vi "ArrayToExcel.vi"() -> ()   [LabVIEW 2020]
uses:
  <vilib>/Analysis/NI_AALBase.lvlib
panel:
  out "F-format string":string[][](array[string])
  out "Waveform Graph":dbl[][](graph)
  # "Diego Jáuregui Ontiveros\nCarlos Uriel Casas Casas\nAlejandro López González"
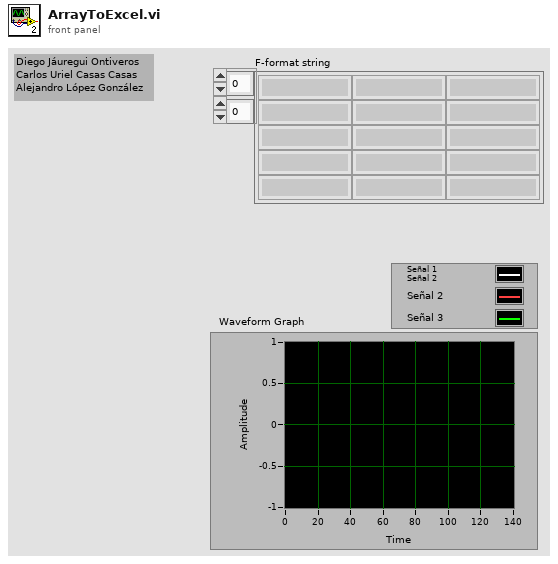
[diagram p1: front panel]
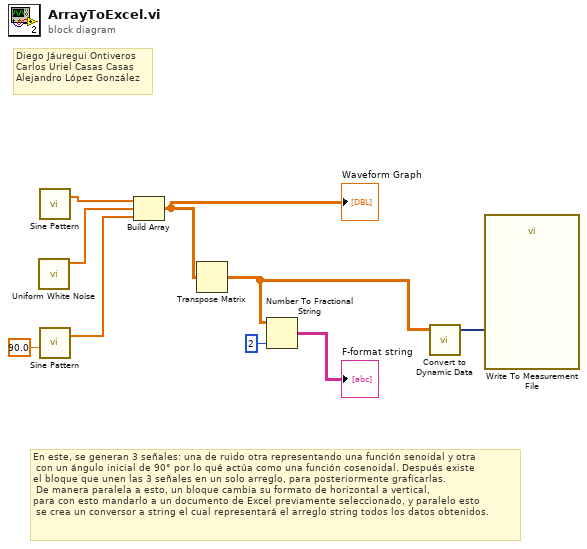
[diagram p0: block diagram]
diagram:
  # "En este, se generan 3 señales: una de ruido otra representando una función senoidal y otra\n con un ángulo inicial de 90° por lo qué actúa como una función cosenoidal. Después existe \nel bloque que unen las 3 señales en un solo arreglo, para posteriormente graficarlas.\n De manera paralela a esto, un bloque cambia su formato de horizontal a vertical, \npara con esto mandarlo a un documento de Excel previamente seleccionado, y paralelo esto\n se crea un conversor a string el cual representará el arreglo string todos los datos obtenidos."
  # "Diego Jáuregui Ontiveros\nCarlos Uriel Casas Casas\nAlejandro López González"
  n1 = call <vilib>:"Uniform White Noise.vi"() -> ("uniform white noise"=w6:dbl[])  [unwired: 10 in, 1 out]
  n2 = call <vilib>:"Sine Pattern.vi"() -> ("Sinusoidal Pattern"=w7:dbl[])  [unwired: 4 in, 1 out]
  n3 = call <vilib>:"Sine Pattern.vi"("phase(degrees)"=90.0) -> ("Sinusoidal Pattern"=w5:dbl[])  [unwired: 3 in, 1 out]
  n4 = Build Array(w7, w6, w5) -> (w2:dbl[][])
  "Waveform Graph" <- w2
  n5 = Transpose Matrix(1:w2) -> (0:w4:dbl[][])
  n6 = Number To Fractional String(number=w4, precision (6)=i16 2) -> (F-format string=→"F-format string":string[][])  [unwired: 2 in]
  n7 = call "Convert to Dynamic Data"("2D Array"=w4) -> ("Dynamic Data Type"=w3:dynamicdata)  [unwired: 3 in]
  n8 = call "Write To Measurement File"("Signals"=w3) -> ()  [unwired: 16 in, 3 out]
